vi "msleep.vi"(11 "milliseconds":cluster{}) -> ()   [LabVIEW 2019, in "apdm.lvlib"]
doc: "APDM_EXPORT void apdm_msleep(const uint64_t milliseconds);"
uses:
  apdm.lvlib
  Lee Lab/CP FES Walking 2018/Code/Working/LabVIEW/apdm.dll
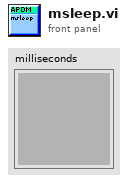
[diagram p1: front panel]
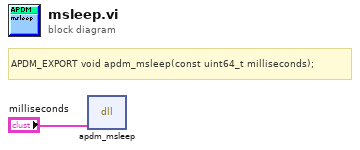
[diagram p0: block diagram]
diagram:
  # "APDM_EXPORT void apdm_msleep(const uint64_t milliseconds);"
  n1 = dll-call lib="C:/Users/jfalesi/Dropbox/Lee Lab/CP FES Walking 2018/Code/Working/LabVIEW/apdm.*" fn="apdm_msleep"("milliseconds"="milliseconds") -> ()  [unwired: 5 in, 2 out]
